vi "TipsDialog.vi"() -> ()   [LabVIEW 2020, in "UmlEditor.lvclass"]
uses:
  <resource>/Framework/Providers/Open_GDS/UML/UmlEditor_class/UmlEditor.lvclass
  <vilib>/Utility/miscctls.llb/LVBoundsTypeDef.ctl
  <resource>/Framework/Providers/Open_GDS/ClassProviders/Common/GdsLanguage/GdsLanguage_LanguageID.ctl
panel:
  out "Tip":i32
  in  "Save":bool
  in  "TipsString":string
  in  "_PreviousTip":bool
  in  "_NextTip":bool
  in  "_DontShowTip":bool
  in  "_Close":bool
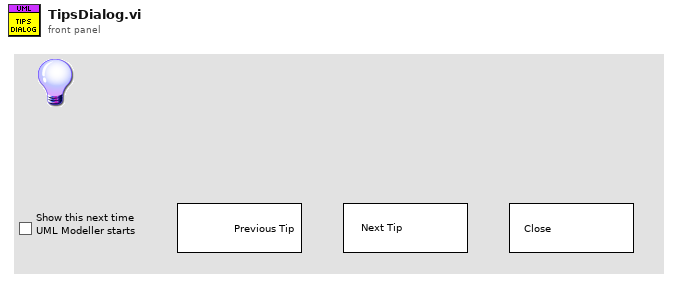
[diagram p1: front panel]
types:
  T1 = typedef "GdsLanguage_ObjectAttributes.ctl" = cluster{"Language":T2, "TranslatedStrings":string[], "StringIDArray":string[], "LanguageFilesDirectory":path, "AvailableLanguages":T2[]}
  T2 = typedef "GdsLanguage_LanguageID.ctl" = enum16{"< undefined >", "aa", "ab", "af", "am", "ar", "as", "ay", "az", "ba", "be", "bg", "bh", "bi", "bn", "bo", "br", "ca", "co", "cs", "cy", "da", "de", "dz", "el", "en", "eo", "es", "et", "eu", "fa", "fi", "fj", "fo", "fr", "fy", "ga", "gd", "gl", "gn", "gu", "gv", "ha", "he", "hi", "hr", "hu", "hy", "ia", "id", "ie", "ik", "is", "it", "iu", "ja", "jv", "ka", "kk", "kl", "km", "kn", "ko", "ks", "ku", "ky", "la", "li", "ln", "lo", "lt", "lv", "mg", "mi", "mk", "ml", "mn", "mo", "mr", "ms", "mt", "my", "na", "ne", "nl", "no", "oc", "om", "or", "pa", "pl", "ps", "pt", "qu", "rm", "rn", "ro", "ru", "rw", "sa", "sd", "sg", "sh", "si", "sk", "sl", "sm", "sn", "so", "sq", "sr", "ss", "st", "su", "sv", "sw", "ta", "te", "tg", "th", "ti", "tk", "tl", "tn", "to", "tr", "ts", "tt", "tw", "ug", "uk", "ur", "uz", "vi", "vo", "wo", "xh", "yi", "yo", "zh", "zu"}
  T3 = typedef "LVBoundsTypeDef.ctl" = cluster{"Width":u32, "Height":u32}
  T4 = typedef "LVRectTypeDef.ctl" = cluster{"Left":i16, "Top":i16, "Right":i16, "Bottom":i16}
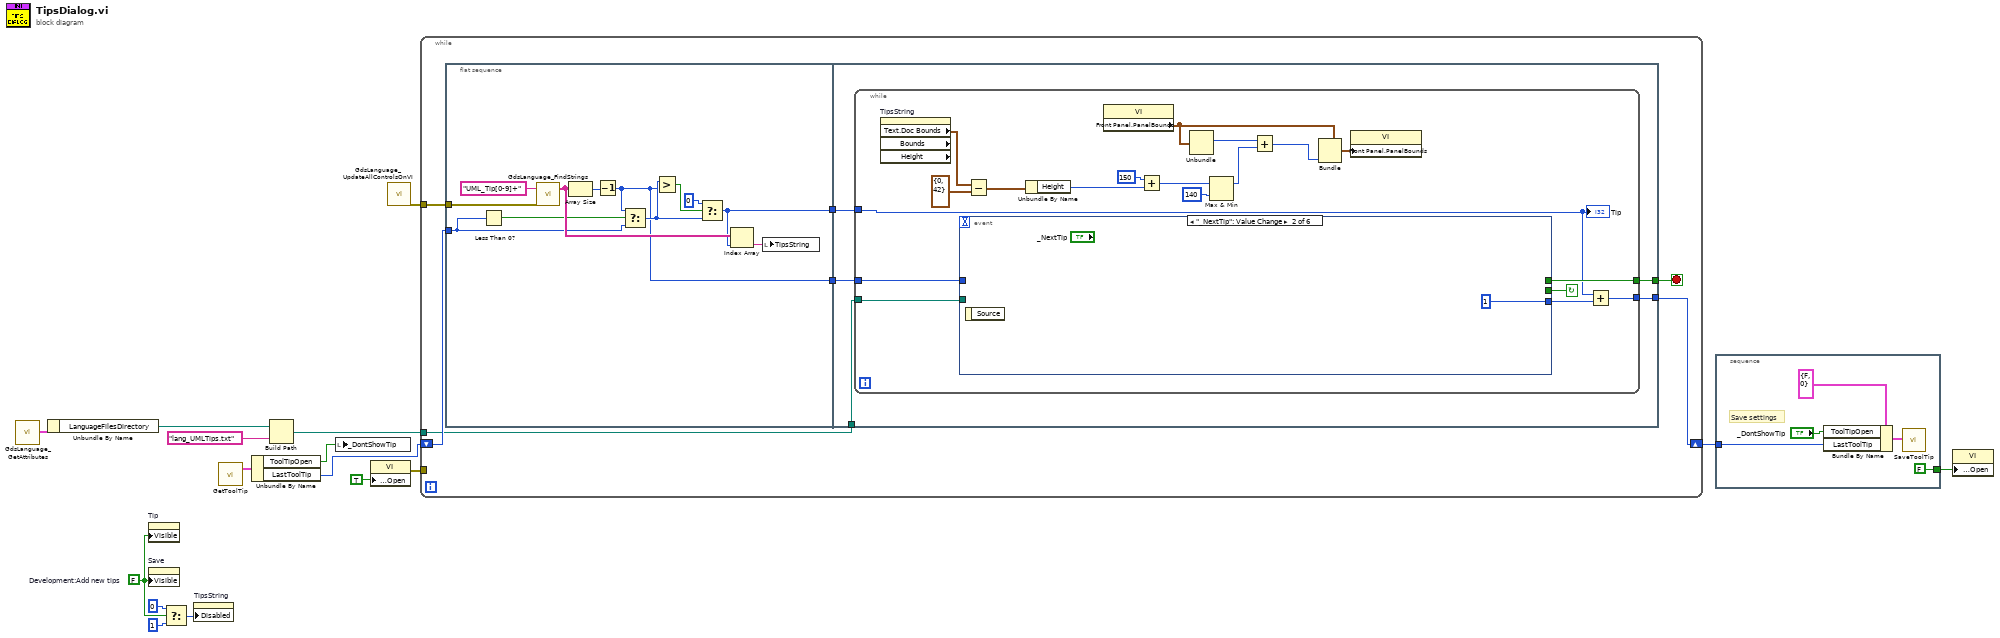
[diagram p0: block diagram]
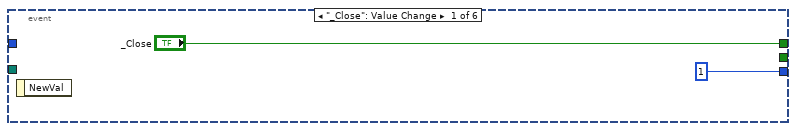
[diagram p2: hidden frame]
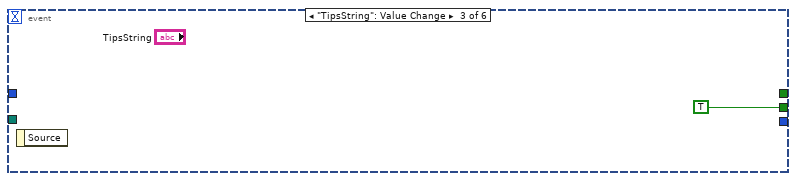
[diagram p3: hidden frame]
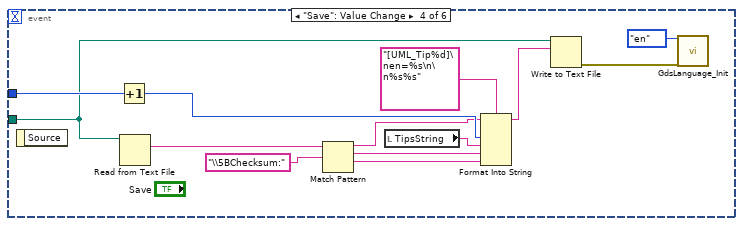
[diagram p4: hidden frame]
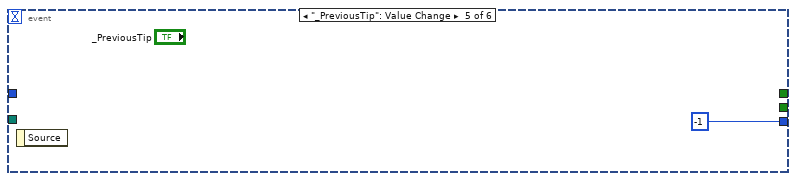
[diagram p5: hidden frame]
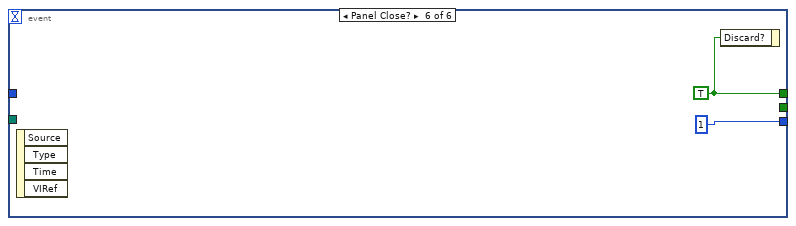
[diagram p6: hidden frame]
diagram:
  w12 = FALSE  # Development:Add new tips
  n1 = call <resource>:"GdsLanguage_GetAttributes.vi"() -> ("Attributes"=w1:T1)  [unwired: 3 in, 16 out]
  n2 = Unbundle By Name(w1) -> ("LanguageFilesDirectory"=w11:path)
  n3 = property on="Tip" class="DigNum (strict)"("Visible"=w12) -> ()  [unwired: 2 in, 2 out]
  n4 = property on="Save" class="Bool"("Visible"=w12) -> ()  [unwired: 2 in, 2 out]
  n5 = Select(t=u8 0 ("Disabled"), s=w12, f=u8 1) -> (s? t:f=w14:u8)
  n6 = property on="TipsString" class="Str"("Disabled"=w14) -> ()  [unwired: 2 in, 2 out]
  n7 = call <resource>:"GetToolTip.vi"() -> ("ToolTip"=w7:cluster{"ToolTipOpen":bool, "LastToolTip":i32})  [unwired: 1 in, 18 out]
  n8 = Unbundle By Name(w7) -> ("ToolTipOpen"=w6:bool, "LastToolTip"=w5:i32)
  n9 = Build Path(base path=w11, name or relative path="lang_UMLTips.txt") -> (appended path=w8:path)
  n10 = local write "_DontShowTip"(w6) -> ()
  n11 = property class="VI"("Front Panel.Open"=TRUE ("Front Panel Window:Open")) -> (error out=w3:errorcluster)  [unwired: 2 in, 1 out]
  n12 = call <resource>:"GdsLanguage_UpdateAllControlsOnVI.vi"() -> ("error out"=w16:errorcluster)  [unwired: 4 in, 15 out]
  n13 = while {
    tunnel: w16 -> [w22]
    shift-right: [w19] -> w9
    shift-left: w5 -> [w21]
    tunnel: w8 -> [w18]
    tunnel: w3 -> [_]
    stop <- w23 stop-if-true
    n14 = flat-sequence {
      tunnel: w22 -> [w35]
      tunnel: w21 -> [w25]
      tunnel: [w27] -> w20
      tunnel: [w24] -> w17
      tunnel: [w40] -> w23
      tunnel: w20 -> [w38]
      tunnel: [w39] -> w19
      tunnel: w18 -> [w37]
      tunnel: w17 -> [w36]
      frame #0 {
        n15 = Less Than 0?(x=w25) -> (x < 0?=w29:bool)
        n16 = call <resource>:"GdsLanguage_FindStrings.vi"("SearchStringPattern"="UML_Tip[0-9]+", "error in (no error)"=w35) -> ("StringsOut"=w33:string[])  [unwired: 17 out]
        n17 = Array Size(array=w33) -> (size(s)=w32:i32)
        n18 = Decrement(x=w32) -> (x-1=w24:i32)
        n19 = Select(t=w24, s=w29, f=w25) -> (s? t:f=w28:i32)
        n20 = Greater?(x=w28, y=w24) -> (0:w31:bool)
        n21 = Select(t=0, s=w31, f=w28) -> (s? t:f=w27:i32)
        n22 = Index Array(array=w33, index=w27) -> (element=w26:string)
        n23 = local write "TipsString"(w26) -> ()
      }
      frame #1 {
        n24 = while {
          tunnel: [w51] -> w40
          tunnel: [w48] -> w39
          tunnel: w38 -> [w47]
          tunnel: w37 -> [w46]
          tunnel: w36 -> [w44]
          stop <- w45 continue-if-true
          n25 = property on="TipsString" class="Str" props=["Text", "Doc Bounds", "Bounds", "Height"]() -> ("Text.Doc Bounds"=w58:T3)  [unwired: 2 in, 4 out]
          n26 = event shown="[1] \"_NextTip\": Value Change" {
            selector: _ -> [_ _ _ _ _ _]
            dyn-events: _ -> [_ _ _ _ _ _]
            timeout: _ -> [_ _ _ _ _ _]
            tunnel: ["_Close" _ _ _ _ w79] -> w51
            tunnel: [1 1 _ _ -1 1] -> w49
            tunnel: w44 -> [_ _ _ w76 _ _]
            tunnel: w46 -> [_ _ _ w67 _ _]
            tunnel: [_ _ TRUE _ _ _] -> w45
            event "_Close": Value Change {
              n27 = event-data() -> ()  [unwired: 2 out]
            }
            event "_NextTip": Value Change {
              n28 = event-data() -> ()  [unwired: 2 out]
            }
            event "TipsString": Value Change {
              n29 = event-data() -> ()  [unwired: 2 out]
            }
            event "Save": Value Change {
              n30 = event-data() -> ()  [unwired: 2 out]
              n31 = Increment(x=w76) -> (x+1=w72:i32)
              n32 = Read from Text File(file (use dialog)=w67) -> (text=w75:string)  [unwired: 1 in, 5 out]
              n33 = Match Pattern(string=w75, regular expression="\\5BChecksum:") -> (before substring=w71:string, match substring=w70:string, after substring=w69:string)  [unwired: 2 out]
              n34 = local read "TipsString"() -> (w64:string)
              n35 = Format Into String(format string="[UML_Tip%d]\nen=%s\n\n%s%s", initial string=w71, w72, w64, w70, w69) -> (resulting string=w68:string)  [unwired: 1 in, 1 out]
              n36 = Write to Text File(file (use dialog)=w67, text=w68) -> (error out=w66:errorcluster)  [unwired: 1 in, 3 out]
              n37 = call <resource>:"GdsLanguage_Init.vi"("PrimaryLanguage"=GdsLanguage_LanguageID."en", "error in (no error)"=w66) -> ()  [unwired: 2 in, 16 out]
            }
            event "_PreviousTip": Value Change {
              n38 = event-data() -> ()  [unwired: 2 out]
            }
            event Panel Close? {
              w79 = TRUE ("Close")
              n39 = event-data() -> ()  [unwired: 5 out]
              n40 = event-data("Discard?"=w79) -> ()  [unwired: 1 in, 1 out]
            }
          }
          n41 = Subtract(x=w58, y=T3 {"Width"=0, "Height"=42} ("Text.Document Bounds")) -> (x-y=w57:T3)
          n42 = Unbundle By Name(w57) -> ("Height"=w53:u32)
          n43 = property class="VI"() -> ("Front Panel.PanelBounds"=w55:T4)  [unwired: 2 in, 2 out]
          n44 = Add(x=u32 150, y=w53) -> (x+y=w43:u32)
          n45 = Unbundle(w55) -> ("Top"=w54:i16)  [unwired: 3 out]
          n46 = Max & Min(x=w43, y=u32 140) -> (max(x,y)=w42:u32)  [unwired: 1 out]
          n47 = Add(x=w54, y=w42) -> (x+y=w52:u32)
          n48 = Bundle(cluster=w55, "Bottom"=w52) -> (w56:T4)  [unwired: 3 out]
          n49 = property class="VI"("Front Panel.PanelBounds"=w56) -> ()  [unwired: 2 in, 2 out]
          n50 = Add(x=w47, y=w49) -> (x+y=w48:i32)
          "Tip" <- w47
        }
      }
    }
  }
  n51 = stacked-sequence {
    tunnel: w9 -> [w84]
    tunnel: [FALSE ("Front Panel Window:Open")] -> w2
    frame #0 {
      # "Save settings"
      n52 = Bundle By Name(cluster=cluster{"ToolTipOpen":bool, "LastToolTip":i32} {"ToolTipOpen"=FALSE, "LastToolTip"=0} ("ToolTip"), "ToolTipOpen"="_DontShowTip", "LastToolTip"=w84) -> (w82:cluster{"ToolTipOpen":bool, "LastToolTip":i32})
      n53 = call <resource>:"SaveToolTip.vi"("ToolTip"=w82) -> ()  [unwired: 1 in, 18 out]
    }
  }
  n54 = property class="VI"("Front Panel.Open"=w2) -> ()  [unwired: 2 in, 2 out]
